vi "plot_query.vi"(6 "Small?":bool, 7 "Selected Dust Events":u64[](array[numeric]), 8 "error in (no error)":errorcluster, 9 "Limit no. of events":u64=10000, 10 "Limited?":bool=TRUE, 11 "Constraints":T1 {"Estimate Quality" scale=0.0..5.0}) -> (0 "error out":errorcluster, 1 "Total Number of triggers":u64, 2 "Number of Matching Events":u64, 3 "Dust Array":T2[](array[typedef]) {"File Location" items=["Unknown"=-1, "Storage"=0, "Processing"=1, "Unmerged"=2]; "Estimate Source" items=["Any Source."=-2, "No Shot"=-1, "Basic Labview Estimate"=0, "IDL Estimate From Andrew"=1, "IDL Estimate From Tobin"=2, "Old Metadata"=3]}, 4 "Dust Info":cluster{"Density":dbl, "Name":string}[](array[cluster]))   [LabVIEW 2013]
doc: "Returns four important pieces of information: an array of dust to be plotted, the number of events being plotted, the total number of triggers, and information about the dust being plotted."
uses:
  <userlib>/Accelerator/User Interface/Controls/Query_Dust_Event.ctl
  <userlib>/Accelerator/User Interface/Controls/Estimate_source.ctl
  <userlib>/Accelerator/User Interface/Controls/File_location.ctl
  <userlib>/Accelerator/User Interface/Controls/Constraints.ctl
  <userlib>/_OpenG.lib/array/array.llb/Sort 1D Array (DBL)__ogtk.vi
  <userlib>/_OpenG.lib/array/array.llb/Empty 1D Array (U64)__ogtk.vi
  <userlib>/_OpenG.lib/array/array.llb/Remove Duplicates from 1D Array (String)__ogtk.vi
  <userlib>/_OpenG.lib/array/array.llb/Delete Elements from 1D Array (DBL)__ogtk.vi
  <vilib>/addons/database/_DB Variant To Data/Database Variant To Data.xnode
panel:
  out "Experiment/Group Limits":string[](array[string])
  out "Quality Limit":string[](array[string])
  out "Velocity/Mass Limits":string[](array[string])
  out "Timestamp Limit":string[](array[string])
  out "Selected Events Syntax":string
  out "Count Events Syntax":string
  out "SQL Query Syntax":string
  # "Dust Event"
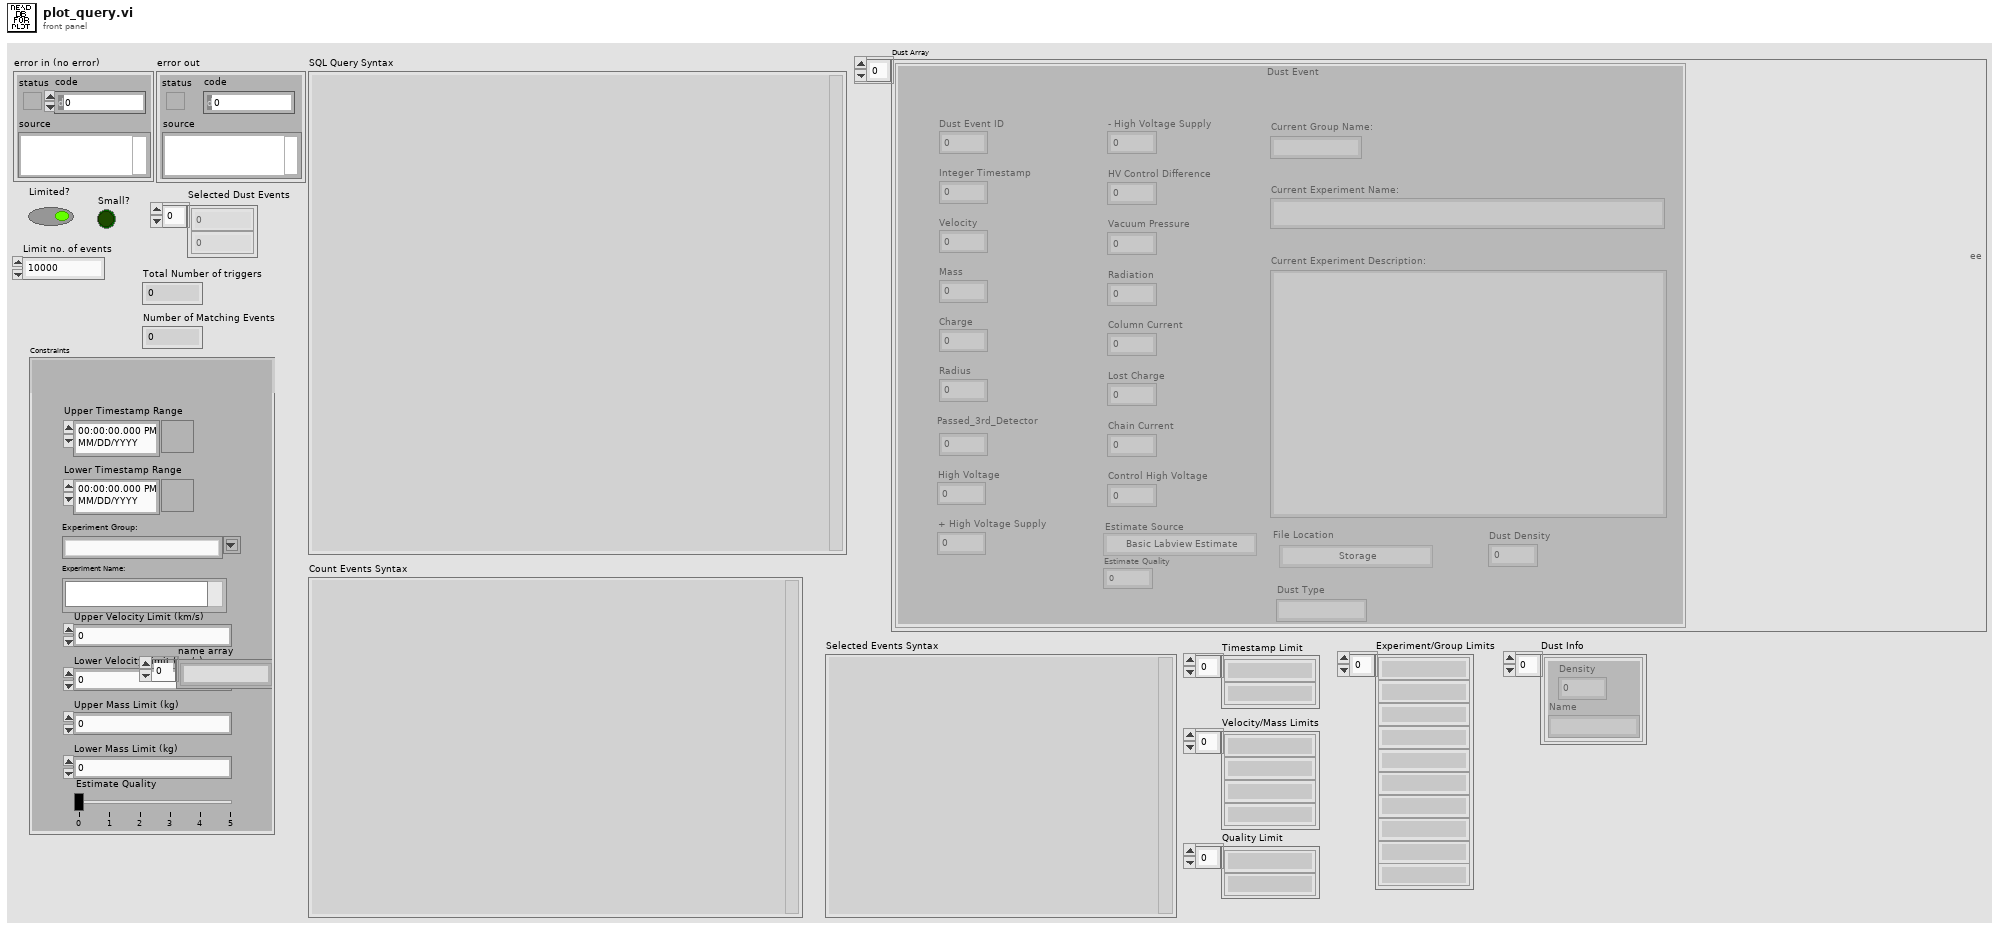
[diagram p1: front panel]
types:
  T1 = typedef "Constraints.ctl" = cluster{"Upper Timestamp Range":timestamp, "Lower Timestamp Range":timestamp, "Experiment Group:":string, "Experiment Name:":i32[], "Upper Velocity Limit (km/s)":dbl, "Lower Velocity Limit (km/s)":dbl, "Upper Mass Limit (kg)":dbl, "Lower Mass Limit (kg)":dbl, "name array":string[], "Estimate Quality":cluster{dbl, dbl}}
  T2 = typedef "Query_Dust_Event.ctl" = cluster{"Dust Event ID":i64, "Integer Timestamp":i64, "Velocity":dbl, "Mass":dbl, "Charge":sgl, "Radius":sgl, "Passed_3rd_Detector":i8, "High Voltage":sgl, "+ High Voltage Supply":sgl, "- High Voltage Supply":sgl, "HV Control Difference":sgl, "Vacuum Pressure":sgl, "Radiation":sgl, "Column Current":sgl, "Lost Charge":sgl, "Chain Current":sgl, "Control High Voltage":sgl, "Current Group Name:":string, "Current Experiment Name:":string, "Current Experiment Description:":string, "Estimate Source":T3, "Estimate Quality":i8, "File Location":T4, "Dust Type":string, "Dust Density":sgl}
  T3 = typedef "Estimate_source.ctl" = i8
  T4 = typedef "File_location.ctl" = i8
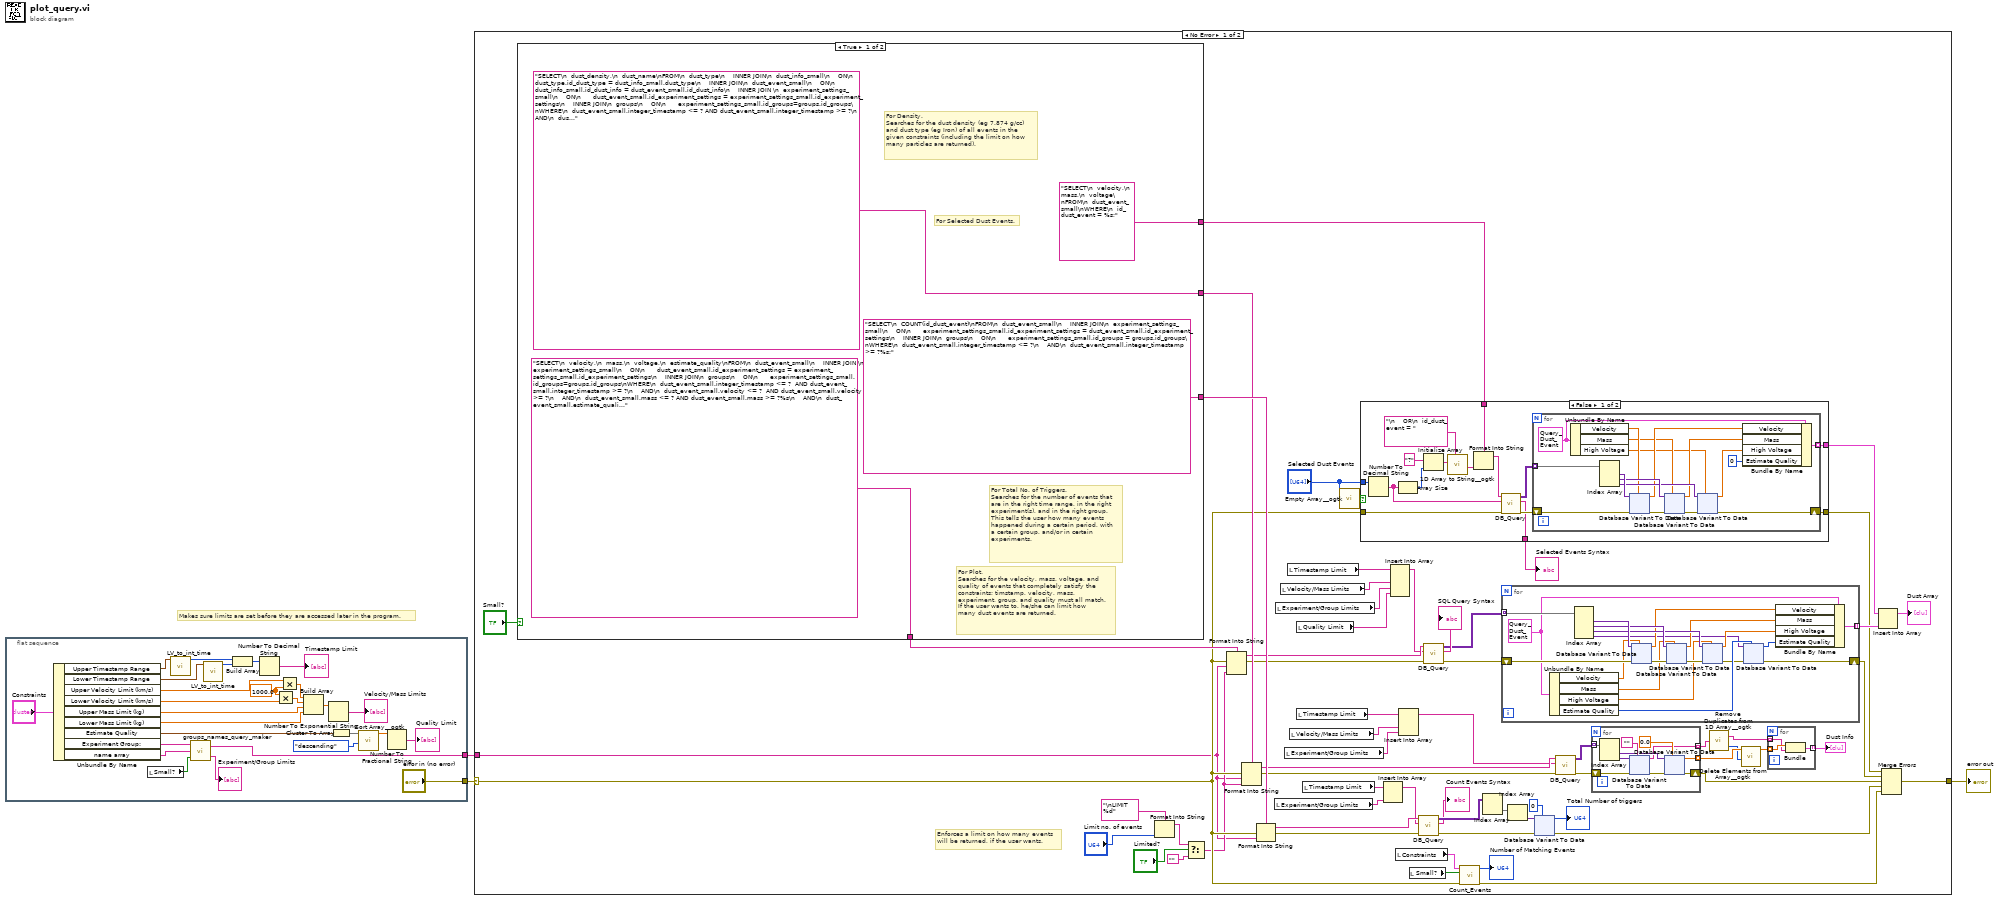
[diagram p0: block diagram]
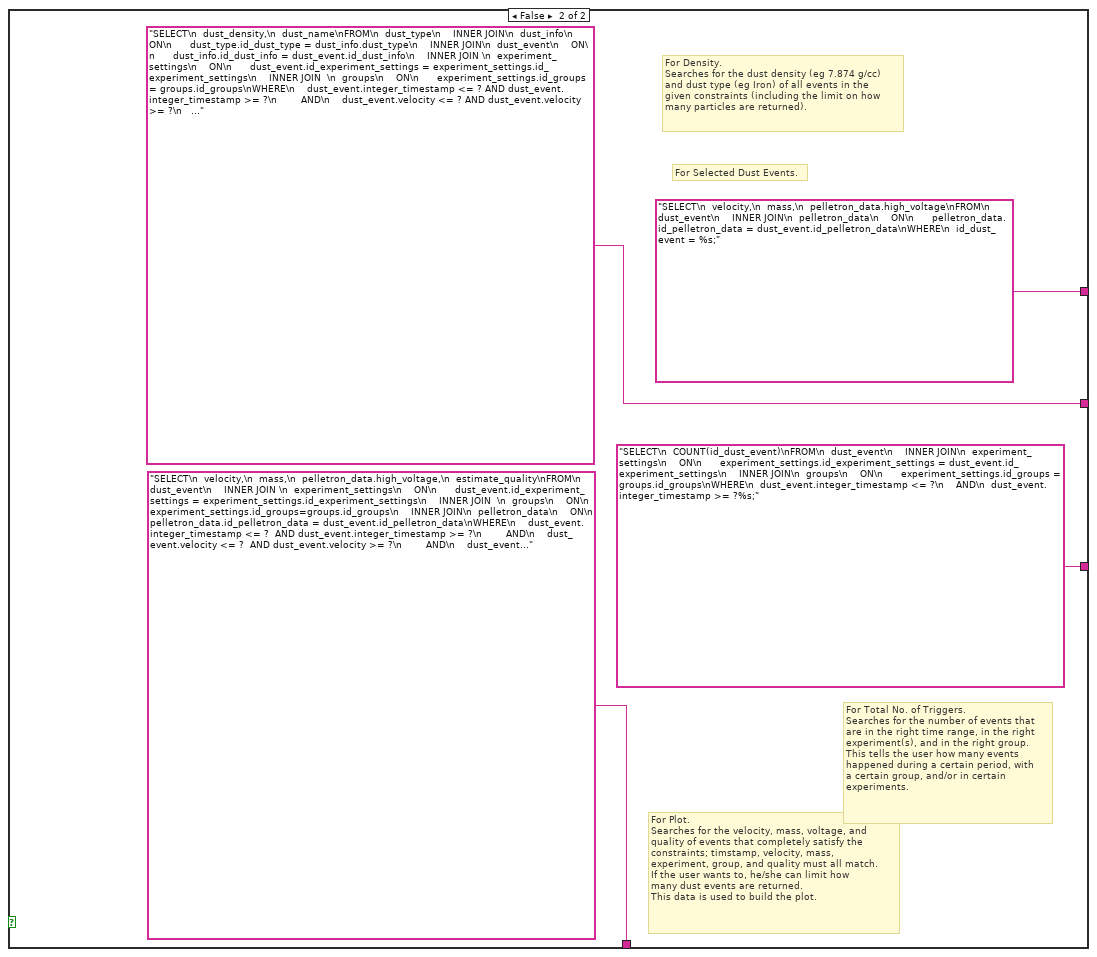
[diagram p3: hidden frame]
diagram:
  # "Makes sure limits are set before they are accessed later in the program."
  n1 = flat-sequence {
    tunnel: ["error in (no error)"] -> w3
    tunnel: [w4] -> w1
    frame #0 {
      w6 = 1000.0 ("y")
      n2 = Unbundle By Name("Constraints") -> ("Upper Timestamp Range"=w7:timestamp, "Lower Timestamp Range"=w8:timestamp, "Upper Velocity Limit (km/s)"=w9:dbl, "Lower Velocity Limit (km/s)"=w10:dbl, "Upper Mass Limit (kg)"=w16:dbl, "Lower Mass Limit (kg)"=w17:dbl, "Estimate Quality"=w22:cluster{dbl, dbl}, "Experiment Group:"=w24:string, "name array"=w25:string[])
      n3 = local read "Small?"() -> (w21:bool)
      n4 = call <userlib>:"LV_to_int_time.vi"("Time Stamp"=w7) -> ("Integer Time"=w12:i64)  [unwired: 8 in, 1 out]
      n5 = call <userlib>:"groups_names_query_maker.vi"("Small?"=w21, "Name Array"=w25, "Group  Name"=w24) -> ("Parameters"=→"Experiment/Group Limits":string[], "Group and Names Query"=w4:string)
      n6 = call <userlib>:"LV_to_int_time.vi"("Time Stamp"=w8) -> ("Integer Time"=w11:i64)  [unwired: 8 in, 1 out]
      n7 = Build Array(w12, w11) -> (w13:i64[])
      n8 = Number To Decimal String(number=w13) -> (decimal integer string=→"Timestamp Limit":string[])  [unwired: 1 in]
      n9 = Multiply(x=w6, y=w10) -> (x*y=w15:dbl)
      n10 = Multiply(x=w9, y=w6) -> (x*y=w14:dbl)
      n11 = Build Array(w14, w15, w16, w17) -> (w18:dbl[])
      n12 = Number To Exponential String(number=w18) -> (E-format string=→"Velocity/Mass Limits":string[])  [unwired: 3 in]
      n13 = Cluster To Array(cluster=w22) -> (array=w23:dbl[])
      n14 = call-poly <userlib>:"Sort Array__ogtk.vi"("Order"=enum16{"ascending", "descending"}."descending", "Array in"=w23) -> ("Sorted Array out"=w20:dbl[])  [unwired: 8 in, 1 out]
      n15 = Number To Fractional String(number=w20) -> (F-format string=→"Quality Limit":string[])  [unwired: 3 in]
    }
  }
  n16 = case shown="No Error" w3 {
    selector: w3 -> [w63 w489]
    tunnel: [w93 w489] -> w2
    tunnel: w1 -> [w39 _]
    frame No Error {
      # "Enforces a limit on how many events\nwill be returned, if the user wants."
      n17 = case shown="True" "Small?" {
        tunnel: ["SELECT\n  velocity,\n  mass,\n  voltage,\n  estimate_quality\nFROM\n  dust_event_small\n    INNER JOIN \n  experiment_settings_small\n    ON\n      dust_event_small.id_experiment_settings = experiment_settings_small.id_experiment_settings\n    INNER JOIN\n  groups\n    ON\n      experiment_settings_small.id_groups=groups.id_groups\nWHERE\n  dust_event_small.integer_timestamp <= ?  AND dust_event_small.integer_timestamp >= ?\n    AND\n  dust_event_small.velocity <= ?  AND dust_event_small.velocity >= ?\n    AND\n  dust_event_small.mass <= ? AND dust_event_small.mass >= ?%s\n    AND\n  dust_event_small.estimate_quality <= ? AND dust_event_small.estimate_quality >= ?\n    AND\n  dust_event_small.estimate_quality > 0\nORDER BY\n  id_dust_event DESC%s;" ("string") "SELECT\n  velocity,\n  mass,\n  pelletron_data.high_voltage,\n  estimate_quality\nFROM\n  dust_event\n    INNER JOIN \n  experiment_settings\n    ON\n      dust_event.id_experiment_settings = experiment_settings.id_experiment_settings\n    INNER JOIN  \n  groups\n    ON\n      experiment_settings.id_groups=groups.id_groups\n    INNER JOIN\n  pelletron_data\n    ON\n      pelletron_data.id_pelletron_data = dust_event.id_pelletron_data\nWHERE\n    dust_event.integer_timestamp <= ?  AND dust_event.integer_timestamp >= ?\n        AND\n    dust_event.velocity <= ?  AND dust_event.velocity >= ?\n        AND\n    dust_event.mass <= ? AND dust_event.mass >= ?%s\n        AND\n    dust_event.estimate_quality <= ? AND dust_event.estimate_quality >= ?\n        AND\n    dust_event.estimate_quality > 0\nORDER BY\n    id_dust_event DESC%s;" ("string")] -> w94
        tunnel: ["SELECT\n  COUNT(id_dust_event)\nFROM\n  dust_event_small\n    INNER JOIN\n  experiment_settings_small\n    ON\n      experiment_settings_small.id_experiment_settings = dust_event_small.id_experiment_settings\n    INNER JOIN\n  groups\n    ON\n      experiment_settings_small.id_groups = groups.id_groups\nWHERE\n  dust_event_small.integer_timestamp <= ?\n    AND\n  dust_event_small.integer_timestamp >= ?%s;" ("SQL query") "SELECT\n  COUNT(id_dust_event)\nFROM\n  dust_event\n    INNER JOIN\n  experiment_settings\n    ON\n      experiment_settings.id_experiment_settings = dust_event.id_experiment_settings\n    INNER JOIN\n  groups\n    ON\n      experiment_settings.id_groups = groups.id_groups\nWHERE\n  dust_event.integer_timestamp <= ?\n    AND\n  dust_event.integer_timestamp >= ?%s;" ("SQL query")] -> w92
        tunnel: ["SELECT\n  dust_density,\n  dust_name\nFROM\n  dust_type\n    INNER JOIN\n  dust_info_small\n    ON\n      dust_type.id_dust_type = dust_info_small.dust_type\n    INNER JOIN\n  dust_event_small\n    ON\n      dust_info_small.id_dust_info = dust_event_small.id_dust_info\n    INNER JOIN \n  experiment_settings_small\n    ON\n      dust_event_small.id_experiment_settings = experiment_settings_small.id_experiment_settings\n    INNER JOIN\n  groups\n    ON\n      experiment_settings_small.id_groups=groups.id_groups\nWHERE\n  dust_event_small.integer_timestamp <= ? AND dust_event_small.integer_timestamp >= ?\n    AND\n  dust_event_small.velocity <= ? AND dust_event_small.velocity >= ?\n    AND\n  dust_event_small.mass <= ? AND dust_event_small.mass >= ?%s\nORDER BY\n  id_dust_event DESC%s; " ("string") "SELECT\n  dust_density,\n  dust_name\nFROM\n  dust_type\n    INNER JOIN\n  dust_info\n    ON\n      dust_type.id_dust_type = dust_info.dust_type\n    INNER JOIN\n  dust_event\n    ON\n      dust_info.id_dust_info = dust_event.id_dust_info\n    INNER JOIN \n  experiment_settings\n    ON\n      dust_event.id_experiment_settings = experiment_settings.id_experiment_settings\n    INNER JOIN  \n  groups\n    ON\n      experiment_settings.id_groups = groups.id_groups\nWHERE\n    dust_event.integer_timestamp <= ? AND dust_event.integer_timestamp >= ?\n        AND\n    dust_event.velocity <= ? AND dust_event.velocity >= ?\n        AND\n    dust_event.mass <= ?  AND dust_event.mass >= ?%s\nORDER BY\n    id_dust_event DESC%s;" ("string")] -> w79
        tunnel: ["SELECT\n  velocity,\n  mass,\n  voltage\nFROM\n  dust_event_small\nWHERE\n  id_dust_event = %s;" "SELECT\n  velocity,\n  mass,\n  pelletron_data.high_voltage\nFROM\n  dust_event\n    INNER JOIN\n  pelletron_data\n    ON\n      pelletron_data.id_pelletron_data = dust_event.id_pelletron_data\nWHERE\n  id_dust_event = %s;"] -> w67
        frame True {
          # "For Selected Dust Events."
          # "For Density.\nSearches for the dust density (eg 7.874 g/cc)\nand dust type (eg Iron) of all events in the\ngiven constraints (including the limit on how\nmany particles are returned)."
          # "For Plot.\nSearches for the velocity, mass, voltage, and\nquality of events that completely satisfy the\nconstraints; timstamp, velocity, mass,\nexperiment, group, and quality must all match.\nIf the user wants to, he/she can limit how\nmany dust events are returned."
          # "For Total No. of Triggers.\nSearches for the number of events that\nare in the right time range, in the right\nexperiment(s), and in the right group.\nThis tells the user how many events\nhappened during a certain period, with\na certain group, and/or in certain\nexperiments."
        }
        frame False {
          # "For Total No. of Triggers.\nSearches for the number of events that\nare in the right time range, in the right\nexperiment(s), and in the right group.\nThis tells the user how many events\nhappened during a certain period, with\na certain group, and/or in certain\nexperiments."
          # "For Selected Dust Events."
          # "For Density.\nSearches for the dust density (eg 7.874 g/cc)\nand dust type (eg Iron) of all events in the\ngiven constraints (including the limit on how\nmany particles are returned)."
          # "For Plot.\nSearches for the velocity, mass, voltage, and\nquality of events that completely satisfy the\nconstraints; timstamp, velocity, mass,\nexperiment, group, and quality must all match.\nIf the user wants to, he/she can limit how\nmany dust events are returned. \nThis data is used to build the plot."
        }
      }
      n18 = Format Into String(format string="\nLIMIT %d", "Limit no. of events") -> (resulting string=w85:string)  [unwired: 2 in, 1 out]
      n19 = Select(t=w85, s="Limited?", f="") -> (s? t:f=w59:string)
      n20 = Format Into String(format string=w94, error in=w63, w39, w59) -> (resulting string=w46:string, error out=w49:errorcluster)  [unwired: 1 in]
      n21 = Format Into String(format string=w79, error in=w63, w39, w59) -> (resulting string=w50:string, error out=w53:errorcluster)  [unwired: 1 in]
      n22 = Format Into String(format string=w92, error in=w63, w39) -> (resulting string=w55:string, error out=w57:errorcluster)  [unwired: 1 in]
      n23 = local read "Experiment/Group Limits"() -> (w42:string[])
      n24 = local read "Experiment/Group Limits"() -> (w35:string[])
      n25 = local read "Velocity/Mass Limits"() -> (w34:string[])
      n26 = local read "Experiment/Group Limits"() -> (w38:string[])
      n27 = local read "Timestamp Limit"() -> (w33:string[])
      n28 = local read "Velocity/Mass Limits"() -> (w40:string[])
      n29 = local read "Quality Limit"() -> (w36:string[])
      n30 = local read "Timestamp Limit"() -> (w44:string[])
      n31 = local read "Timestamp Limit"() -> (w43:string[])
      n32 = call-poly <userlib>:"Empty Array__ogtk.vi"("Array"="Selected Dust Events") -> ("Empty Array?"=w60:bool)  [unwired: 8 in]
      n33 = case shown="False" w60 {
        tunnel: "Selected Dust Events" -> [w109 _]
        tunnel: w67 -> [w106 _]
        tunnel: [w105 _] -> w66
        tunnel: w63 -> [w96 w223]
        tunnel: [w104 w223] -> w62
        tunnel: [w95 _] -> w31
        frame False {
          n34 = Number To Decimal String(number=w109) -> (decimal integer string=w97:string[])  [unwired: 1 in]
          n35 = Array Size(array=w97) -> (size(s)=w99:i32)
          n36 = Initialize Array("?", w99) -> (w101:string[])
          n37 = call <userlib>:"1D Array to String__ogtk.vi"("delimiter (Tab)"="\n    OR\n  id_dust_event = ", "Array of Strings"=w101) -> ("delimited string"=w107:string)  [unwired: 9 in]
          n38 = Format Into String(format string=w106, w107) -> (resulting string=w98:string)  [unwired: 2 in, 1 out]
          n39 = call <userlib>:"DB_Query.vi"("error in (no error)"=w96, "Parameters"=w97, "Parameterized Query"=w98) -> ("error out"=w102:errorcluster, "Query in Standard Format"=w95:string, "Results"=w103:variant[][])  [unwired: 6 in]
          n40 = for {
            tunnel: [w125] -> w105 mode=indexing
            tunnel: w103 -> [w120] mode=indexing
            shift-right: [w121] -> w104
            shift-left: w102 -> [w124]
            w126 = T2 {"Dust Event ID"=0, "Integer Timestamp"=0, "Velocity"=0.0, "Mass"=0.0, "Charge"=0.0, "Radius"=0.0, "Passed_3rd_Detector"=0, "High Voltage"=0.0, "+ High Voltage Supply"=0.0, "- High Voltage Supply"=0.0, "HV Control Difference"=0.0, "Vacuum Pressure"=0.0, "Radiation"=0.0, "Column Current"=0.0, "Lost Charge"=0.0, "Chain Current"=0.0, "Control High Voltage"=0.0, "Current Group Name:"="", "Current Experiment Name:"="", "Current Experiment Description:"="", "Estimate Source"=0, "Estimate Quality"=0, "File Location"=0, "Dust Type"="", "Dust Density"=0.0} ("Cluster")
            n41 = Unbundle By Name(w126) -> ("Velocity"=w116:dbl, "Mass"=w114:dbl, "High Voltage"=w112:sgl)
            n42 = Index Array(array=w120) -> (element #1=w119:variant, element #2=w118:variant, element #3=w117:variant)  [unwired: 3 in]
            n43 = xnode "Database Variant To Data"("database variant"=w119, "error in (no error)"=w124, "type"=w116) -> ("data"=w115:dbl, "error out"=w123:errorcluster)
            n44 = xnode "Database Variant To Data"("database variant"=w118, "error in (no error)"=w123, "type"=w114) -> ("data"=w113:dbl, "error out"=w122:errorcluster)
            n45 = xnode "Database Variant To Data"("database variant"=w117, "error in (no error)"=w122, "type"=w112) -> ("data"=w111:sgl, "error out"=w121:errorcluster)
            n46 = Bundle By Name(cluster=w126, "Velocity"=w115, "Mass"=w113, "High Voltage"=w111, "Estimate Quality"=i8 0) -> (w125:T2)
          }
        }
        frame True {
        }
      }
      "Selected Events Syntax" <- w31
      n47 = Insert Into Array(array=w43, new element=w42) -> (w41:string[])  [unwired: 1 in]
      n48 = Insert Into Array(array=w33, new element #1=w34, new element #2=w35, new element #3=w36) -> (w32:string[])  [unwired: 1 in]
      n49 = local read "Constraints"() -> (w70:T1)
      n50 = Insert Into Array(array=w44, new element #1=w40, new element #2=w38) -> (w37:string[])  [unwired: 1 in]
      n51 = local read "Small?"() -> (w71:bool)
      n52 = call <userlib>:"DB_Query.vi"("error in (no error)"=w57, "Parameters"=w41, "Parameterized Query"=w55) -> ("error out"=w56:errorcluster, "Query in Standard Format"=→"Count Events Syntax":string, "Results"=w58:variant[][])  [unwired: 6 in]
      n53 = call <userlib>:"DB_Query.vi"("error in (no error)"=w49, "Parameters"=w32, "Parameterized Query"=w46) -> ("error out"=w45:errorcluster, "Query in Standard Format"=→"SQL Query Syntax":string, "Results"=w47:variant[][])  [unwired: 6 in]
      n54 = call <userlib>:"Count_Events.vi"("error in (no error)"=w63, "Small?"=w71, "Constraints"=w70) -> ("error out"=w68:errorcluster, "Number of Events"=→"Number of Matching Events":u64)  [unwired: 7 in]
      n55 = Index Array(array=w58) -> (element=w91:variant[])  [unwired: 2 in]
      n56 = for {
        tunnel: w47 -> [w360] mode=indexing
        shift-right: [w352] -> w83
        shift-left: w45 -> [w359]
        tunnel: [w351] -> w65 mode=indexing
        w357 = T2 {"Dust Event ID"=0, "Integer Timestamp"=0, "Velocity"=0.0, "Mass"=0.0, "Charge"=0.0, "Radius"=0.0, "Passed_3rd_Detector"=0, "High Voltage"=0.0, "+ High Voltage Supply"=0.0, "- High Voltage Supply"=0.0, "HV Control Difference"=0.0, "Vacuum Pressure"=0.0, "Radiation"=0.0, "Column Current"=0.0, "Lost Charge"=0.0, "Chain Current"=0.0, "Control High Voltage"=0.0, "Current Group Name:"="", "Current Experiment Name:"="", "Current Experiment Description:"="", "Estimate Source"=0, "Estimate Quality"=0, "File Location"=0, "Dust Type"="", "Dust Density"=0.0} ("Cluster")
        n57 = Unbundle By Name(w357) -> ("Velocity"=w350:dbl, "Mass"=w348:dbl, "High Voltage"=w346:sgl, "Estimate Quality"=w344:i8)
        n58 = Index Array(array=w360) -> (element #1=w358:variant, element #2=w356:variant, element #3=w354:variant, element #4=w341:variant)  [unwired: 4 in]
        n59 = xnode "Database Variant To Data"("database variant"=w358, "error in (no error)"=w359, "type"=w350) -> ("data"=w349:dbl, "error out"=w355:errorcluster)
        n60 = xnode "Database Variant To Data"("database variant"=w356, "error in (no error)"=w355, "type"=w348) -> ("data"=w347:dbl, "error out"=w353:errorcluster)
        n61 = xnode "Database Variant To Data"("database variant"=w354, "error in"=w353, "type"=w346) -> ("data"=w345:sgl, "error out"=w342:errorcluster)
        n62 = xnode "Database Variant To Data"("database variant"=w341, "error in (no error)"=w342, "type"=w344) -> ("data"=w343:i8, "error out"=w352:errorcluster)
        n63 = Bundle By Name(cluster=w357, "Velocity"=w349, "Mass"=w347, "High Voltage"=w345, "Estimate Quality"=w343) -> (w351:T2)
      }
      n64 = Index Array(array=w91) -> (element=w90:variant)  [unwired: 1 in]
      n65 = xnode "Database Variant To Data"("database variant"=w90, "error in (no error)"=w56, "type"=u64 0) -> ("data"=→"Total Number of triggers":u64, "error out"=w82:errorcluster)
      n66 = call <userlib>:"DB_Query.vi"("error in (no error)"=w53, "Parameters"=w37, "Parameterized Query"=w50) -> ("error out"=w52:errorcluster, "Results"=w51:variant[][])  [unwired: 6 in, 1 out]
      n67 = for {
        tunnel: w51 -> [w244] mode=indexing
        shift-right: [w237] -> w81
        shift-left: w52 -> [w239]
        tunnel: [w236] -> w77 mode=indexing
        tunnel: [w235] -> w76 mode=indexing
        n68 = Index Array(array=w244) -> (element #1=w240:variant, element #2=w243:variant)  [unwired: 2 in]
        n69 = xnode "Database Variant To Data"("database variant"=w243, "error in (no error)"=w239, "type"="") -> ("data"=w236:string, "error out"=w238:errorcluster)
        n70 = xnode "Database Variant To Data"("database variant"=w240, "error in (no error)"=w238, "type"=0.0) -> ("data"=w235:dbl, "error out"=w237:errorcluster)
      }
      n71 = call-poly <userlib>:"Remove Duplicates from 1D Array__ogtk.vi"("Input Array"=w77) -> ("Output Array"=w73:string[], "indices of removed elements"=w75:i32[])
      n72 = call-poly <userlib>:"Delete Elements from Array__ogtk.vi"("indices"=w75, "array"=w76) -> ("array w/ subset deleted"=w74:dbl[])  [unwired: 8 in, 1 out]
      n73 = for {
        tunnel: w74 -> [w226] mode=indexing
        tunnel: w73 -> [w225] mode=indexing
        tunnel: [w224] -> w72 mode=indexing
        n74 = Bundle(w226, "String"=w225) -> (w224:cluster{dbl, "String":string})  [unwired: 1 in]
      }
      "Dust Info" <- w72
      n75 = Insert Into Array(array=w66, new element=w65) -> (→"Dust Array":T2[])  [unwired: 1 in]
      n76 = Merge Errors(w62, w83, w81, w82, w68) -> (w93:errorcluster)
    }
    frame Error {
    }
  }
  "error out" <- w2
